vi "Broadcast Sonicator Settings.vi"(8 "error in (no error)":errorcluster, 10 "Message Queues":T5, 11 "Scale Module Config":T1={"GUID"="", "Drop Coords"={"Horizontal"=0, "Vertical"=0}, "Process Name"="", "Queue Name"="", "Settings"={"Cycle Period"=500.0, "Sonicator Type"="", "SS P100 Settings"={"VISA resource name"="", "Simulated?"=FALSE}, "Setpoint (µm)"=0.0, "Cutoff (W)"=0.0}, "Load Count"=0}) -> (0 "error out":errorcluster)   [LabVIEW 2018, in "Sonicator Module.lvlib"]
uses:
  Sonicator Module.lvlib
  Sonicator Message Queues.ctl
  support/Message Queue/Message Cluster.ctl
  Controls/Sonicator Module Config Cluster.ctl
  <vilib>/Utility/miscctls.llb/LVPoint32TypeDef.ctl
  Controls/Sonicator Module Settings Cluster.ctl
  Sonic Systems P100/Sonic Systems P100 Settings.ctl
  support/Message Queue/Enqueue Message (Single).vi
  support/Message Queue/Message Queue.lvlib
  Sonic Systems P100/Sonic Systems P100.lvlib
panel:
  # "Sonicator Settings"
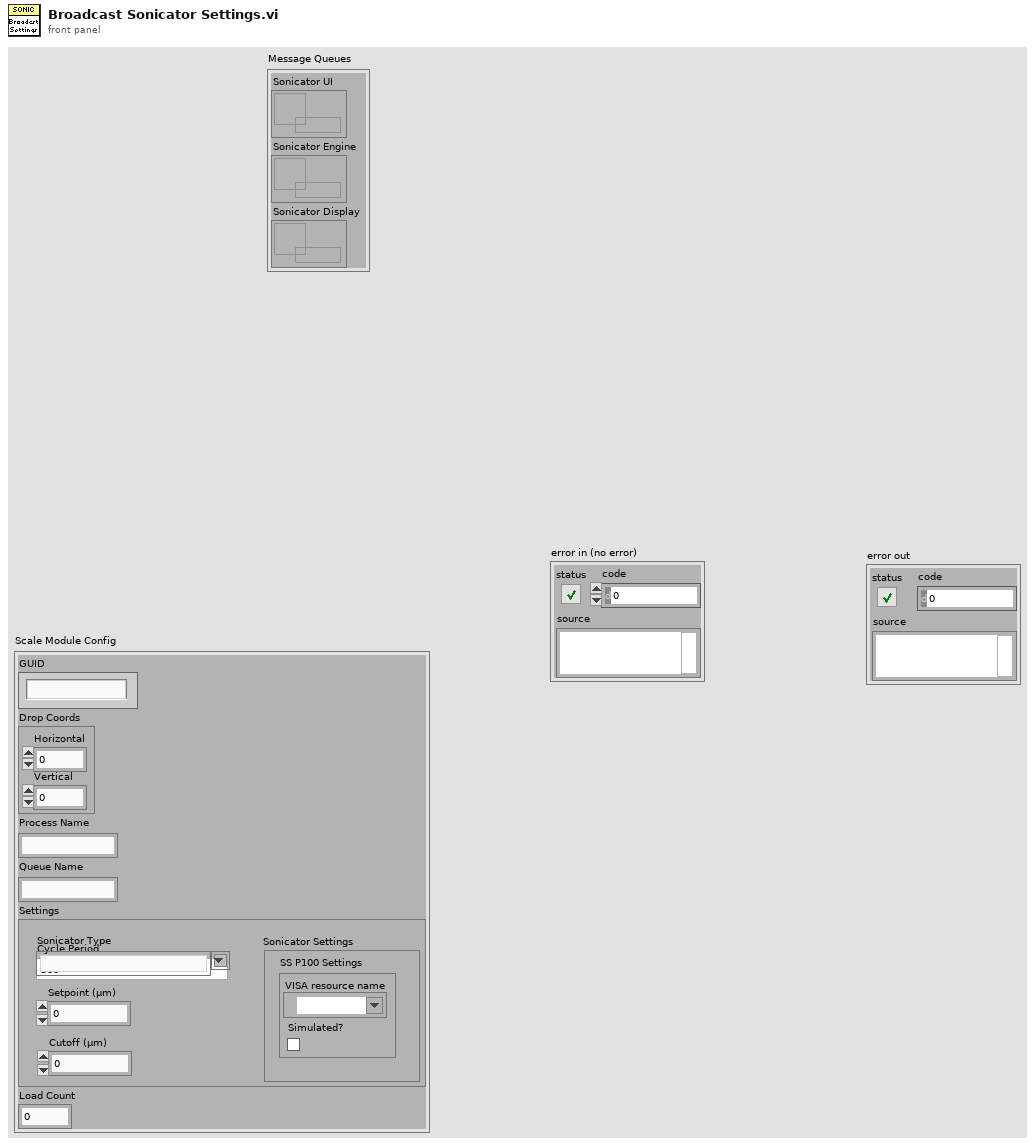
[diagram p1: front panel]
types:
  T1 = typedef "Sonicator Module.lvlib/Sonicator Module Config Cluster.ctl" = cluster{"GUID":string, "Drop Coords":T2, "Process Name":string, "Queue Name":string, "Settings":T3, "Load Count":i32}
  T2 = typedef "LVPoint32TypeDef.ctl" = cluster{"Horizontal":i32, "Vertical":i32}
  T3 = typedef "Sonicator Module.lvlib/Sonicator Module Settings Cluster.ctl" = cluster{"Cycle Period":dbl, "Sonicator Type":string, "SS P100 Settings":T4, "Setpoint (µm)":dbl, "Cutoff (W)":dbl}
  T4 = typedef "Sonic Systems P100.lvlib/Sonic Systems P100 Settings.ctl" = cluster{"VISA resource name":refnum<visa-resource-name>, "Simulated?":bool}
  T5 = typedef "Sonicator Module.lvlib/Sonicator Message Queues.ctl" = cluster{"Sonicator UI":refnum<queue>, "Sonicator Engine":refnum<queue>, "Sonicator Display":refnum<queue>}
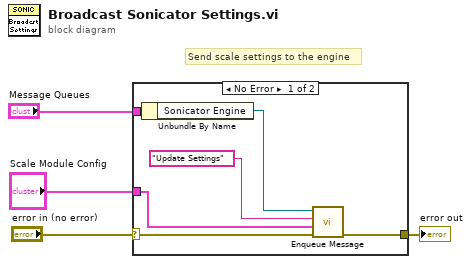
[diagram p0: block diagram]
diagram:
  # "Send scale settings to the engine"
  n1 = case shown="No Error" "error in (no error)" {
    selector: "error in (no error)" -> [w6 w11]
    tunnel: [w5 w11] -> w2
    tunnel: "Scale Module Config" -> [w8 _]
    tunnel: "Message Queues" -> [w10 _]
    frame No Error {
      n2 = Unbundle By Name(w10) -> ("Sonicator Engine"=w9:refnum<queue>)
      n3 = call-poly "Enqueue Message.vi"("error in (no error)"=w6, "Message Data"=w8, "Message"="Update Settings", "Message Queue"=w9) -> ("error out"=w5:errorcluster)  [unwired: 6 in, 1 out]
    }
    frame Error {
    }
  }
  "error out" <- w2
